vi "cSM Default Error Handler.vi"(8 "States in":string[](array[string]), 11 "error in (no error)":errorcluster) -> (0 "States out":string[](array[string]), 3 "error out":errorcluster)   [LabVIEW 2021, in "EDT VIE.lvlib"]
uses:
  EDT VIE.lvlib
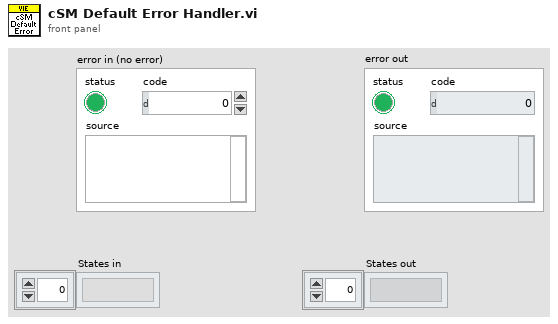
[diagram p1: front panel]
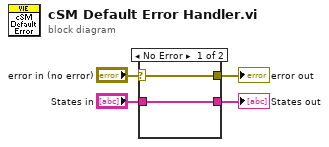
[diagram p0: block diagram]
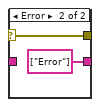
[diagram p2: hidden frame]
diagram:
  n1 = case shown="No Error" "error in (no error)" {
    selector: "error in (no error)" -> [w6 w7]
    tunnel: [w6 w7] -> w3
    tunnel: [w5 string[] ["Error"] ("t")] -> w2
    tunnel: "States in" -> [w5 _]
    frame No Error {
    }
    frame Error {
    }
  }
  "States out" <- w2
  "error out" <- w3
